vi "Main.vi"(11 "Module Admin":refnum<class "Delacor_lib_QMH_Cloneable Module Admin.lvclass">) -> ()   [LabVIEW 2020, in "Interfase.lvlib"]
doc: "This template is based off of the Queued Message Handler design pattern and the Queued Message Handler project template that ships with LabVIEW.\n\nThe main difference is that the queue is private to this module and communication between modules is performed via Broadcast and Request events.\n\nRequest events are wrapped in public API methods and are handled in the Event Handling Loop (EHL) of this VI. Any module can register for Broadcast events sent by this module. The EHL generates messages based on user interface actions.\n\nThe Message Handling Loop (MHL) processes messages generated by the EHL, or by other messages. The messages are string values, so new messages can be added easily to the Message Cases case structure in the MHL. Each message cluster can also provide an optional value for Message Data, which is a variant that can be converted to whatever message-specific data is required.\n_____\nBased on Delacor QMH Project Template 5.0.0.82."
uses:
  Interfase.lvlib
  <vilib>/Delacor/Delacor QMH/Libraries/Cloneable Module Admin_class/Delacor_lib_QMH_Cloneable Module Admin.lvclass
  C:/Program Files/National Instruments/LabVIEW 2020/vi.lib/Delacor/Delacor QMH/Libraries/Module Admin_class/Delacor_lib_QMH_Module Admin.lvclass
  Controles/Brand combobox.ctl
  Module Data--cluster.ctl
  <vilib>/Delacor/Delacor QMH/Libraries/Cloneable Module Admin_class/Delacor_lib_QMH_Cloneable Module Admin.lvclass/Delacor_lib_QMH_Cloneable Module Admin.ctl
  Stop Argument--cluster.ctl
  <vilib>/Delacor/Delacor QMH/Libraries/Message Queue_class/Delacor_lib_QMH_Message Queue.lvclass/Delacor_lib_QMH_Message Queue.ctl
  <vilib>/Delacor/Delacor QMH/Libraries/Module Admin_class/Delacor_lib_QMH_Module Admin.lvclass/Delacor_lib_QMH_Module Admin.ctl
  Read ADC Argument--cluster.ctl
  Set Port Status Argument--cluster.ctl
  Get Port Status Argument--cluster.ctl
  Set Pin Argument--cluster.ctl
  Get Pin Status Argument--cluster.ctl
  Implementations/Simulado/Simulado.lvclass
  C:/Users/deLili/Desktop/UDLSB IET/701/Instrumentacion Virtual/Fork/Proyecto 7mo/Proyecto-7mo-IV/Abstract/Serial device/Serial device.lvclass
  Implementations/NXP/NXP.lvclass
  Implementations/Cypress/Cypress.lvclass
  <vilib>/Delacor/Delacor QMH/Libraries/Cloneable Module Admin_class/Delacor_lib_QMH_Get Module ID.vi
  <vilib>/Delacor/Delacor QMH/Libraries/Message Queue_class/Delacor_lib_QMH_Enqueue Message (Single).vi
  <vilib>/Delacor/Delacor QMH/Libraries/Module Admin_class/Delacor_lib_QMH_Get External Launch.vi
  <vilib>/Utility/error.llb/Error Cluster From Error Code.vi
  <vilib>/ErrorRing/Error Ring.xnode
  <vilib>/Delacor/Delacor QMH/Libraries/Message Queue_class/Delacor_lib_QMH_Message Queue.lvclass
  Abstract/Serial device/Serial device.lvclass
panel:
  in  "Visa Com Port":refnum<visa-resource-name>
  in  "Serial Device Brand":T1
  in  "Configure serial device":bool
  out "RESPUESTA":string
  in  "Get Pin":bool
  out "Pin Value":bool
  in  "Pin":dbl
  in  "Port":dbl
  in  "Set Port":bool
  in  "Value":string
  in  "Port":dbl
  in  "Get Port":bool
  out "Port Value":bool[](array[boolean])
  in  "Port":dbl
  in  "Set Pin":bool
  in  "Value":bool
  in  "Pin":dbl
  in  "Port":dbl
  in  "Read ADC":bool
  out "error out":errorcluster
  in  "Channel":dbl
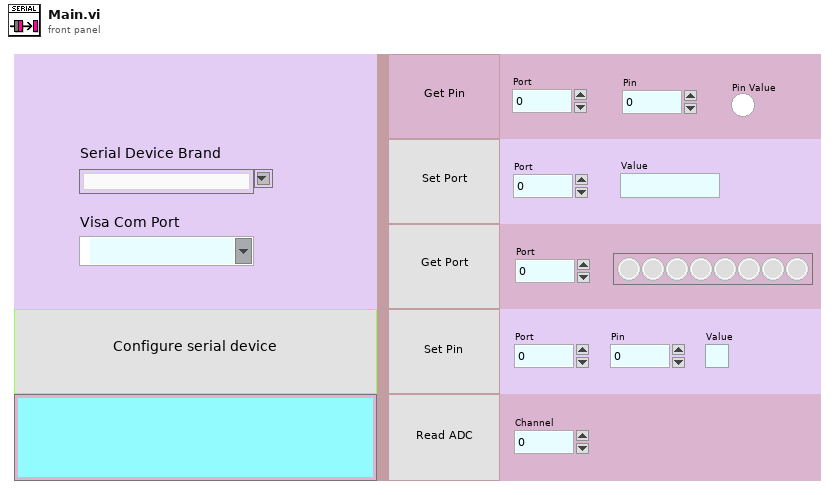
[diagram p1: front panel]
types:
  T1 = typedef "Serial device.lvclass/Brand combobox.ctl" = string
  T2 = typedef "Interfase.lvlib/Request Events--cluster.ctl" = cluster{"Stop Module":refnum<user-event>, "Show Panel":refnum<user-event>, "Hide Panel":refnum<user-event>, "Show Diagram":refnum<user-event>, "Get Module Execution Status":refnum<user-event>, "Read ADC":refnum<user-event>, "Set Port Status":refnum<user-event>, "Get Port Status":refnum<user-event>, "Set Pin":refnum<user-event>, "Get Pin Status":refnum<user-event>}
  T3 = typedef "Interfase.lvlib/Module Data--cluster.ctl" = cluster{"Status":string}
  T4 = enum32{"invalid lock state", "Not Locked", "Locked (No Password)", "Password-protected"}
  T5 = typedef "Interfase.lvlib/Stop Argument--cluster.ctl" = cluster{"Module ID":i32, "Origin":string, "Exit via Stop Module Req?":bool, "Wait for Module to stop?":bool}
  T6 = typedef "Interfase.lvlib/Read ADC Argument--cluster.ctl" = cluster{"Module ID":i32, "Channel":dbl}
  T7 = typedef "Interfase.lvlib/Set Port Status Argument--cluster.ctl" = cluster{"Module ID":i32, "Port":dbl, "Value":string}
  T8 = typedef "Interfase.lvlib/Get Port Status Argument--cluster.ctl" = cluster{"Module ID":i32, "Port":dbl}
  T9 = typedef "Interfase.lvlib/Set Pin Argument--cluster.ctl" = cluster{"Module ID":i32, "Port":dbl, "Pin":dbl, "Value":bool}
  T10 = typedef "Interfase.lvlib/Get Pin Status Argument--cluster.ctl" = cluster{"Module ID":i32, "Port":dbl, "Pin":dbl, "Pin Value":bool}
  T11 = enum32{"Invalid", "Standard", "Closed", "Hidden", "Minimized", "Maximized"}
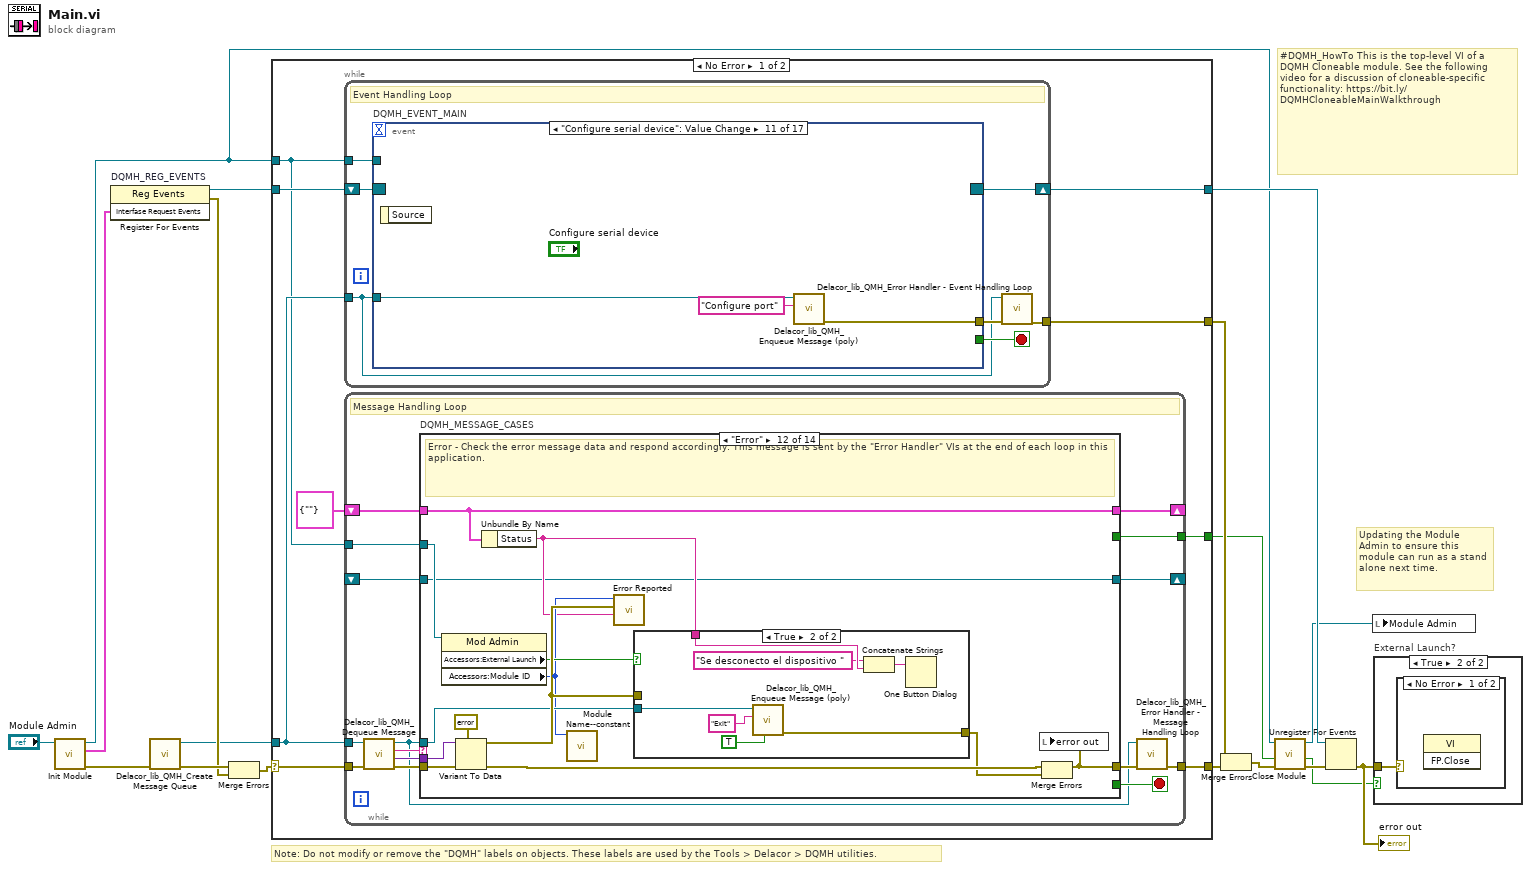
[diagram p0: block diagram]
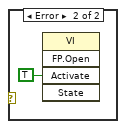
[diagram p3: hidden frame]
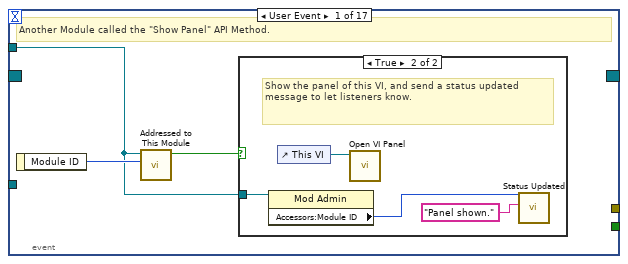
[diagram p4: hidden frame]
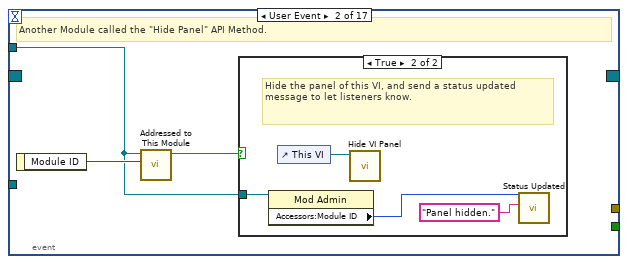
[diagram p6: hidden frame]
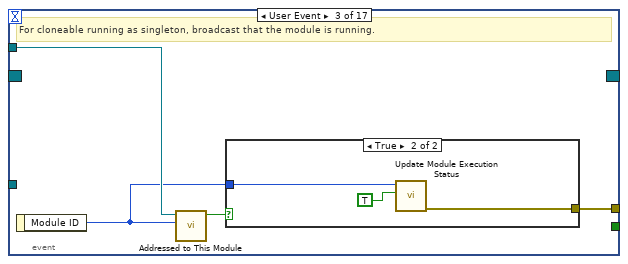
[diagram p8: hidden frame]
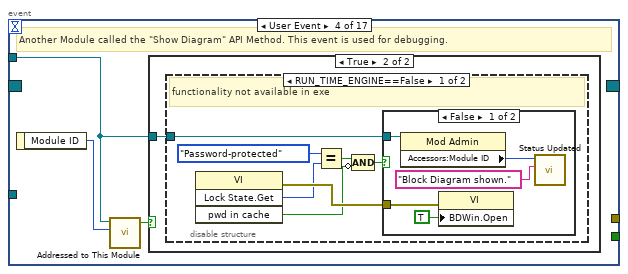
[diagram p10: hidden frame]
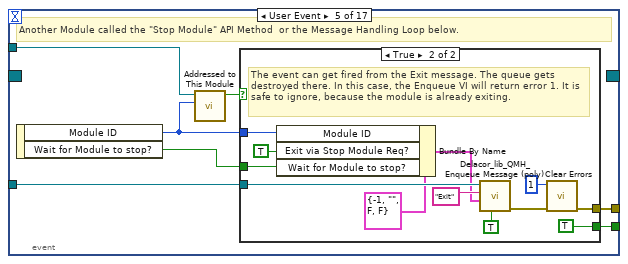
[diagram p14: hidden frame]
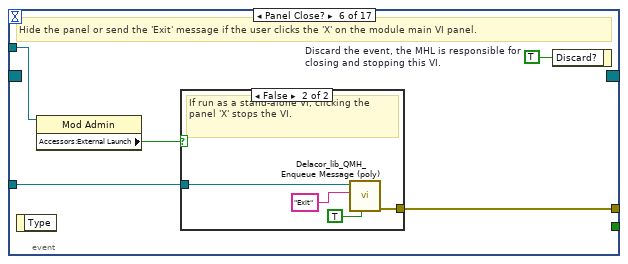
[diagram p16: hidden frame]
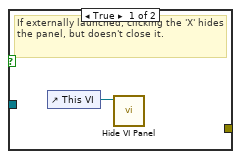
[diagram p17: hidden frame]
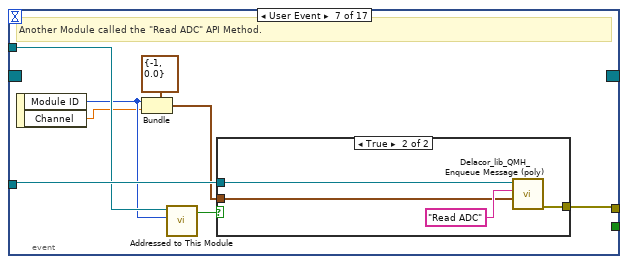
[diagram p18: hidden frame]
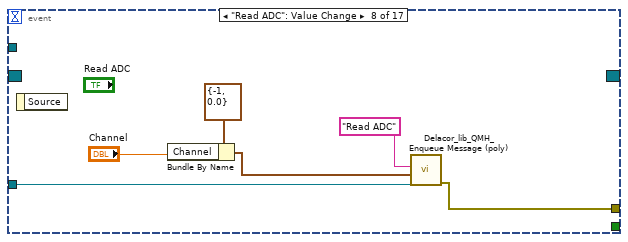
[diagram p20: hidden frame]
diagram:
  # "#DQMH_HowTo This is the top-level VI of a DQMH Cloneable module. See the following video for a discussion of cloneable-specific functionality: https://bit.ly/DQMHCloneableMainWalkthrough"
  # "Note: Do not modify or remove the \"DQMH\" labels on objects. These labels are used by the Tools > Delacor > DQMH utilities."
  # "Updating the Module Admin to ensure this module can run as a stand alone next time."
  n1 = call "Init Module.vi"("Cloneable Module Admin in"="Module Admin") -> ("error out"=w15:errorcluster, "Interfase Request Events"=w7:T2, "Cloneable Module Admin out"=w4:refnum<class "Delacor_lib_QMH_Cloneable Module Admin.lvclass">)  [unwired: 8 in]
  n2 = register-events "DQMH_REG_EVENTS"(w7) -> (reference out=w8:refnum<event-registration>, error out=w10:errorcluster)  [unwired: 2 in]
  n3 = call <vilib>:"Delacor_lib_QMH_Create Message Queue.vi"("error in (no error)"=w15) -> ("error out"=w12:errorcluster, "Message Queue"=w6:refnum<class "Delacor_lib_QMH_Message Queue.lvclass">)  [unwired: 9 in]
  n4 = Merge Errors(w12, w10) -> (w11:errorcluster)
  n5 = case shown="No Error" w11 {
    selector: w11 -> [w25 w419]
    tunnel: [w27 w418] -> w16
    tunnel: [w24 w426] -> w9
    tunnel: w8 -> [w22 w426]
    tunnel: w6 -> [w21 w417]
    tunnel: [w26 _] -> w17
    tunnel: w4 -> [w20 w422]
    tunnel: [w19 _] -> w2
    frame No Error {
      n6 = while {
        tunnel: w21 -> [w28]
        shift-right: [w31] -> w24
        shift-left: w22 -> [w32]
        tunnel: [w33] -> w26
        tunnel: w20 -> [w29]
        stop <- w30 stop-if-true
        # "Event Handling Loop"
        n7 = event "DQMH_EVENT_MAIN" shown="[10] \"Configure serial device\": Value Change" {
          selector: w32 -> [_ _ _ _ _ _ _ _ _ _ _ _ _ _ _ _ _]
          dyn-events: [_ _ _ _ _ _ _ _ _ _ _ _ _ _ _ _ _] -> w31
          timeout: _ -> [_ _ _ _ _ _ _ _ _ _ _ _ _ _ _ _ _]
          tunnel: [_ _ _ _ w74 _ _ _ _ _ _ _ _ _ _ _ _] -> w30
          tunnel: w28 -> [_ _ _ _ w77 w92 w108 w114 w127 w135 w141 w149 w157 w169 w179 w191 w201]
          tunnel: [_ _ w52 _ w78 w95 w101 w113 w119 w132 w140 w142 w156 w160 w180 w182 w196] -> w34
          tunnel: w29 -> [w35 w42 w50 w56 w76 w93 w106 _ w125 _ _ w147 _ w167 _ w189 _]
          event User Event {
            # "Another Module called the \"Show Panel\" API Method."
            n8 = event-data() -> ("Module ID"=w36:i32)  [unwired: 1 in]
            n9 = call "Addressed to This Module.vi"("Module ID from Argument"=w36, "Module Admin"=w35) -> ("Addressed to this instance?"=w37:bool)  [unwired: 8 in, 1 out]
            n10 = case shown="True" w37 {
              tunnel: w35 -> [_ w39]
              frame False {
              }
              frame True {
                # "Show the panel of this VI, and send a status updated message to let listeners know."
                n11 = property class="Mod Admin"(reference=w39) -> ("Accessors:Module ID"=w38:i32)  [unwired: 1 in, 2 out]
                n12 = control-ref of="This VI"() -> (w41:refnum<vi>)
                n13 = call "Open VI Panel.vi"("VI"=w41) -> ()  [unwired: 10 in, 1 out]
                n14 = call "Status Updated.vi"("Status"="Panel shown." ("format string"), "Module ID"=w38) -> ()  [unwired: 9 in, 1 out]
              }
            }
          }
          event User Event {
            # "Another Module called the \"Hide Panel\" API Method."
            n15 = event-data() -> ("Module ID"=w43:i32)  [unwired: 1 in]
            n16 = call "Addressed to This Module.vi"("Module ID from Argument"=w43, "Module Admin"=w42) -> ("Addressed to this instance?"=w44:bool)  [unwired: 8 in, 1 out]
            n17 = case shown="True" w44 {
              tunnel: w42 -> [_ w46]
              frame False {
              }
              frame True {
                # "Hide the panel of this VI, and send a status updated message to let listeners know."
                n18 = property class="Mod Admin"(reference=w46) -> ("Accessors:Module ID"=w45:i32)  [unwired: 1 in, 2 out]
                n19 = control-ref of="This VI"() -> (w48:refnum<vi>)
                n20 = call "Hide VI Panel.vi"("VI"=w48) -> ()  [unwired: 10 in, 1 out]
                n21 = call "Status Updated.vi"("Status"="Panel hidden." ("format string"), "Module ID"=w45) -> ()  [unwired: 9 in, 1 out]
              }
            }
          }
          event User Event {
            # "For cloneable running as singleton, broadcast that the module is running."
            n22 = event-data() -> ("Module ID"=w49:i32)  [unwired: 1 in]
            n23 = call "Addressed to This Module.vi"("Module ID from Argument"=w49, "Module Admin"=w50) -> ("Addressed to this instance?"=w51:bool)  [unwired: 8 in, 1 out]
            n24 = case shown="True" w51 {
              tunnel: [_ w55] -> w52
              tunnel: w49 -> [_ w54]
              frame False {
              }
              frame True {
                n25 = call "Update Module Execution Status.vi"("Running?"=TRUE, "Module ID"=w54) -> ("error out"=w55:errorcluster)  [unwired: 9 in]
              }
            }
          }
          event User Event {
            # "Another Module called the \"Show Diagram\" API Method. This event is used for debugging."
            n26 = event-data() -> ("Module ID"=w57:i32)  [unwired: 1 in]
            n27 = call "Addressed to This Module.vi"("Module ID from Argument"=w57, "Module Admin"=w56) -> ("Addressed to this instance?"=w58:bool)  [unwired: 8 in, 1 out]
            n28 = case shown="True" w58 {
              tunnel: w56 -> [_ w59]
              frame False {
              }
              frame True {
                n29 = disable-structure shown="RUN_TIME_ENGINE==False" {
                  disable-tunnel: w59 -> [w60 _]
                  frame condition #0 (active) {
                    # "functionality not available in exe"
                    n30 = invoke class="VI" method="Lock State.Get"() -> (error out=w66:errorcluster, "Get Lock State"=w65:T4, "pwd in cache"=w62:bool)  [unwired: 4 in, 1 out]
                    n31 = Equal?(x=T4."Password-protected", y=w65) -> (x = y?=w63:bool)
                    n32 = Compound Arithmetic op=AND(w63, invert w62) -> (w61:bool)
                    n33 = case shown="False" w61 {
                      tunnel: w66 -> [w71 _]
                      tunnel: w60 -> [w68 _]
                      frame False {
                        n34 = property class="Mod Admin"(reference=w68) -> ("Accessors:Module ID"=w67:i32)  [unwired: 1 in, 2 out]
                        n35 = property class="VI"(error in=w71, "BDWin.Open"=TRUE ("Block Diagram Window:Open")) -> ()  [unwired: 1 in, 2 out]
                        n36 = call "Status Updated.vi"("Status"="Block Diagram shown." ("format string"), "Module ID"=w67) -> ()  [unwired: 9 in, 1 out]
                      }
                      frame True {
                        # "Password-protected VI, and the password is not in the cache. Do not show the diagram."
                      }
                    }
                  }
                  frame condition #1 {
                  }
                }
              }
            }
          }
          event User Event {
            # "Another Module called the \"Stop Module\" API Method  or the Message Handling Loop below."
            n37 = event-data() -> ("Module ID"=w72:i32, "Wait for Module to stop?"=w73:bool)  [unwired: 1 in]
            n38 = call "Addressed to This Module.vi"("Module ID from Argument"=w72, "Module Admin"=w76) -> ("Addressed to this instance?"=w75:bool)  [unwired: 8 in, 1 out]
            n39 = case shown="True" w75 {
              tunnel: [_ w89] -> w78
              tunnel: w77 -> [_ w85]
              tunnel: [_ TRUE] -> w74
              tunnel: w73 -> [_ w80]
              tunnel: w72 -> [_ w82]
              frame False {
              }
              frame True {
                # "The event can get fired from the Exit message. The queue gets destroyed there. In this case, the Enqueue VI will return error 1. It is safe to ignore, because the module is already exiting."
                n40 = Bundle By Name(cluster=T5 {"Module ID"=-1, "Origin"="", "Exit via Stop Module Req?"=FALSE, "Wait for Module to stop?"=FALSE} ("Stop Argument"), "Module ID"=w82, "Exit via Stop Module Req?"=TRUE, "Wait for Module to stop?"=w80) -> (w79:T5)
                n41 = call-poly <vilib>:"Delacor_lib_QMH_Enqueue Message (poly).vi"("Priority Message? (F)"=TRUE, "Message Data"=w79, "Message"="Exit", "Message Queue in"=w85) -> ("error out"=w90:errorcluster)  [unwired: 6 in, 1 out]
                n42 = call <vilib>:"Clear Errors.vi"("error in (no error)"=w90, "specific error code to clear (0: all)"=1) -> ("error out"=w89:errorcluster)  [unwired: 4 in, 1 out]
              }
            }
          }
          event Panel Close? {
            w94 = TRUE  # Discard the event, the MHL is responsible for closing and stopping this VI.
            # "Hide the panel or send the 'Exit' message if the user clicks the 'X' on the module main VI panel."
            n43 = event-data() -> ()  [unwired: 1 in, 1 out]
            n44 = property class="Mod Admin"(reference=w93) -> ("Accessors:External Launch"=w91:bool)  [unwired: 1 in, 2 out]
            n45 = case shown="False" w91 {
              tunnel: w92 -> [_ w99]
              tunnel: [_ w100] -> w95
              frame True {
                # "If externally launched, clicking the 'X' hides the panel, but doesn't close it."
                n46 = control-ref of="This VI"() -> (w96:refnum<vi>)
                n47 = call "Hide VI Panel.vi"("VI"=w96) -> ()  [unwired: 10 in, 1 out]
              }
              frame False {
                # "If run as a stand-alone VI, clicking the panel 'X' stops the VI."
                n48 = call-poly <vilib>:"Delacor_lib_QMH_Enqueue Message (poly).vi"("Priority Message? (F)"=TRUE, "Message"="Exit", "Message Queue in"=w99) -> ("error out"=w100:errorcluster)  [unwired: 7 in, 1 out]
              }
            }
            n49 = event-data("Discard?"=w94) -> ()  [unwired: 1 in, 1 out]
          }
          event User Event {
            # "Another Module called the \"Read ADC\" API Method."
            n50 = event-data() -> ("Module ID"=w103:i32, "Channel"=w102:dbl)  [unwired: 1 in]
            n51 = Bundle(cluster=T6 {"Module ID"=-1, "Channel"=0.0} ("Read ADC Argument"), "Module ID"=w103, "Channel"=w102) -> (w104:T6)
            n52 = call "Addressed to This Module.vi"("Module ID from Argument"=w103, "Module Admin"=w106) -> ("Addressed to this instance?"=w107:bool)  [unwired: 8 in, 1 out]
            n53 = case shown="True" w107 {
              tunnel: w108 -> [_ w112]
              tunnel: w104 -> [_ w110]
              tunnel: [_ w109] -> w101
              frame False {
              }
              frame True {
                n54 = call-poly <vilib>:"Delacor_lib_QMH_Enqueue Message (poly).vi"("Message Data"=w110, "Message"="Read ADC", "Message Queue in"=w112) -> ("error out"=w109:errorcluster)  [unwired: 7 in, 1 out]
              }
            }
          }
          event "Read ADC": Value Change {
            n55 = event-data() -> ()  [unwired: 1 in, 1 out]
            n56 = Bundle By Name(cluster=T6 {"Module ID"=-1, "Channel"=0.0} ("Read ADC Argument"), "Channel"="Channel") -> (w116:T6)
            n57 = call-poly <vilib>:"Delacor_lib_QMH_Enqueue Message (poly).vi"("Message Data"=w116, "Message"="Read ADC", "Message Queue in"=w114) -> ("error out"=w113:errorcluster)  [unwired: 7 in, 1 out]
          }
          event User Event {
            # "Another Module called the \"Set Port Status\" API Method."
            n58 = event-data() -> ("Module ID"=w122:i32, "Port"=w121:dbl, "Value"=w120:string)  [unwired: 1 in]
            n59 = Bundle(cluster=T7 {"Module ID"=-1, "Port"=0.0, "Value"=""} ("Set Port Status Argument"), "Module ID"=w122, "Port"=w121, "Value"=w120) -> (w123:T7)
            n60 = call "Addressed to This Module.vi"("Module ID from Argument"=w122, "Module Admin"=w125) -> ("Addressed to this instance?"=w126:bool)  [unwired: 8 in, 1 out]
            n61 = case shown="True" w126 {
              tunnel: w127 -> [_ w131]
              tunnel: w123 -> [_ w129]
              tunnel: [_ w128] -> w119
              frame False {
              }
              frame True {
                n62 = call-poly <vilib>:"Delacor_lib_QMH_Enqueue Message (poly).vi"("Message Data"=w129, "Message"="Set Port Status", "Message Queue in"=w131) -> ("error out"=w128:errorcluster)  [unwired: 7 in, 1 out]
              }
            }
          }
          event "Set Port": Value Change {
            n63 = event-data() -> ()  [unwired: 1 in, 1 out]
            n64 = Bundle By Name(cluster=T7 {"Module ID"=-1, "Port"=0.0, "Value"=""} ("Set Port Status Argument"), "Port"="Port", "Value"="Value") -> (w136:T7)
            n65 = call-poly <vilib>:"Delacor_lib_QMH_Enqueue Message (poly).vi"("Message Data"=w136, "Message"="Set Port Status", "Message Queue in"=w135) -> ("error out"=w132:errorcluster)  [unwired: 7 in, 1 out]
          }
          event "Configure serial device": Value Change {
            n66 = event-data() -> ()  [unwired: 1 in, 1 out]
            n67 = call-poly <vilib>:"Delacor_lib_QMH_Enqueue Message (poly).vi"("Message"="Configure port", "Message Queue in"=w141) -> ("error out"=w140:errorcluster)  [unwired: 8 in, 1 out]
          }
          event User Event {
            # "Another Module called the \"Get Port Status\" API Method."
            n68 = event-data() -> ("Module ID"=w144:i32, "Port"=w143:dbl)  [unwired: 1 in]
            n69 = Bundle(cluster=T8 {"Module ID"=-1, "Port"=0.0} ("Get Port Status Argument"), "Module ID"=w144, "Port"=w143) -> (w145:T8)
            n70 = call "Addressed to This Module.vi"("Module ID from Argument"=w144, "Module Admin"=w147) -> ("Addressed to this instance?"=w148:bool)  [unwired: 8 in, 1 out]
            n71 = case shown="True" w148 {
              tunnel: w149 -> [_ w153]
              tunnel: w145 -> [_ w151]
              tunnel: [_ w150] -> w142
              frame False {
              }
              frame True {
                n72 = call-poly <vilib>:"Delacor_lib_QMH_Enqueue Message (poly).vi"("Message Data"=w151, "Message"="Get Port Status", "Message Queue in"=w153) -> ("error out"=w150:errorcluster)  [unwired: 7 in, 1 out]
              }
            }
          }
          event "Get Port": Value Change {
            n73 = event-data() -> ()  [unwired: 1 in, 1 out]
            n74 = Bundle By Name(cluster=T8 {"Module ID"=-1, "Port"=0.0} ("Get Port Status Argument"), "Port"="Port") -> (w155:T8)
            n75 = call-poly <vilib>:"Delacor_lib_QMH_Enqueue Message (poly).vi"("Message Data"=w155, "Message"="Get Port Status", "Message Queue in"=w157) -> ("error out"=w156:errorcluster)  [unwired: 7 in, 1 out]
          }
          event User Event {
            # "Another Module called the \"Set Pin\" API Method."
            n76 = event-data() -> ("Module ID"=w164:i32, "Port"=w163:dbl, "Pin"=w162:dbl, "Value"=w161:bool)  [unwired: 1 in]
            n77 = Bundle(cluster=T9 {"Module ID"=-1, "Port"=0.0, "Pin"=0.0, "Value"=FALSE} ("Set Pin Argument"), "Module ID"=w164, "Port"=w163, "Pin"=w162, "Value"=w161) -> (w165:T9)
            n78 = call "Addressed to This Module.vi"("Module ID from Argument"=w164, "Module Admin"=w167) -> ("Addressed to this instance?"=w168:bool)  [unwired: 8 in, 1 out]
            n79 = case shown="True" w168 {
              tunnel: w169 -> [_ w173]
              tunnel: w165 -> [_ w171]
              tunnel: [_ w170] -> w160
              frame False {
              }
              frame True {
                n80 = call-poly <vilib>:"Delacor_lib_QMH_Enqueue Message (poly).vi"("Message Data"=w171, "Message"="Set Pin", "Message Queue in"=w173) -> ("error out"=w170:errorcluster)  [unwired: 7 in, 1 out]
              }
            }
          }
          event "Set Pin": Value Change {
            n81 = event-data() -> ()  [unwired: 1 in, 1 out]
            n82 = Bundle By Name(cluster=T9 {"Module ID"=-1, "Port"=0.0, "Pin"=0.0, "Value"=FALSE} ("Set Pin Argument"), "Port"="Port", "Pin"="Pin", "Value"="Value") -> (w177:T9)
            n83 = call-poly <vilib>:"Delacor_lib_QMH_Enqueue Message (poly).vi"("Message Data"=w177, "Message"="Set Pin", "Message Queue in"=w179) -> ("error out"=w180:errorcluster)  [unwired: 7 in, 1 out]
          }
          event User Event {
            # "Another Module called the \"Get Pin Status\" API Method."
            n84 = event-data() -> ("Module ID"=w186:i32, "Port"=w185:dbl, "Pin"=w184:dbl, "Pin Value"=w183:bool)  [unwired: 1 in]
            n85 = Bundle(cluster=T10 {"Module ID"=-1, "Port"=0.0, "Pin"=0.0, "Pin Value"=FALSE} ("Get Pin Status Argument"), "Module ID"=w186, "Port"=w185, "Pin"=w184, "Pin Value"=w183) -> (w187:T10)
            n86 = call "Addressed to This Module.vi"("Module ID from Argument"=w186, "Module Admin"=w189) -> ("Addressed to this instance?"=w190:bool)  [unwired: 8 in, 1 out]
            n87 = case shown="True" w190 {
              tunnel: w191 -> [_ w195]
              tunnel: w187 -> [_ w193]
              tunnel: [_ w192] -> w182
              frame False {
              }
              frame True {
                n88 = call-poly <vilib>:"Delacor_lib_QMH_Enqueue Message (poly).vi"("Message Data"=w193, "Message"="Get Pin Status", "Message Queue in"=w195) -> ("error out"=w192:errorcluster)  [unwired: 7 in, 1 out]
              }
            }
          }
          event "Get Pin": Value Change {
            n89 = event-data() -> ()  [unwired: 1 in, 1 out]
            n90 = Bundle By Name(cluster=T10 {"Module ID"=-1, "Port"=0.0, "Pin"=0.0, "Pin Value"=FALSE} ("Get Pin Status Argument"), "Port"="Port", "Pin"="Pin") -> (w197:T10)
            n91 = call-poly <vilib>:"Delacor_lib_QMH_Enqueue Message (poly).vi"("Message Data"=w197, "Message"="Get Pin Status", "Message Queue in"=w201) -> ("error out"=w196:errorcluster)  [unwired: 7 in, 1 out]
          }
        }
        n92 = call-dynamic "Delacor_lib_QMH_Error Handler - Event Handling Loop.vi"("error in (no error)"=w34, "Message Queue in"=w28) -> ("dup error in"=w33:errorcluster)  [unwired: 8 in, 1 out]
      }
      n93 = while {
        tunnel: w21 -> [w208]
        shift-right: [w212] -> _
        shift-left: T3 {"Status"=""} ("Data Cluster") -> [w213]
        tunnel: w25 -> [w216]
        tunnel: [w214] -> w27
        tunnel: w20 -> [w206]
        tunnel: [w205] -> w19
        shift-right: [w204] -> _
        shift-left: _ -> [w203]
        stop <- w211 stop-if-true
        # "Message Handling Loop"
        n94 = call-dynamic "Delacor_lib_QMH_Dequeue Message.vi"("error in (no error)"=w216, "Message Queue in"=w208) -> ("error out"=w215:errorcluster, "Message Data"=w209:variant, "Message"=w210:string, "Message Queue out"=w207:refnum<class "Delacor_lib_QMH_Message Queue.lvclass">)  [unwired: 6 in]
        n95 = case "DQMH_MESSAGE_CASES" shown="\"Error\"" w210 {
          selector: w210 -> [_ _ _ _ _ _ _ _ _ _ _ _ _ w404]
          tunnel: w207 -> [_ _ _ w255 _ w282 _ w321 _ _ _ w360 w393 _]
          tunnel: w215 -> [w234 w244 w253 w270 w277 w295 w312 w331 w348 w352 w355 w368 w399 w406]
          tunnel: [w232 w244 w253 w257 w275 w285 w301 w319 w336 w351 w355 w364 w396 w407] -> w217
          tunnel: w213 -> [w225 w240 w252 w269 w276 w294 w311 w330 w347 w350 w354 w358 w392 w405]
          tunnel: [w225 w239 w252 w269 w276 w294 w311 w330 w347 w350 w354 w358 w392 w405] -> w212
          tunnel: [_ _ _ _ _ _ _ _ _ _ _ _ w391 _] -> w211
          tunnel: w209 -> [_ _ _ w268 w274 w292 w309 w328 w345 _ _ w363 w389 _]
          tunnel: w206 -> [w220 _ _ _ _ _ _ _ _ _ _ w362 w385 w402]
          tunnel: [_ _ _ _ _ _ _ _ _ _ _ _ w387 _] -> w205
          tunnel: [w218 w237 w251 w254 w271 w281 w303 w323 w340 w349 w353 w356 w382 w400] -> w204
          tunnel: w203 -> [w218 _ w251 w265 w271 w289 w305 w322 w341 w349 w353 w356 w383 w400]
          frame "Initialize" {
            # "Initialize - Any operation that needs to be done before the module can receive messages. Synchronize Caller Events.vi will inform Start Module.vi that the module has launched and is ready to receive messages. Module Did Init.vi will broadcast that the module initialized."
            n96 = call "Synchronize Caller Events.vi"("error in (no error)"=w234, "Module Admin"=w220) -> ("error out"=w233:errorcluster, "Module Admin out"=w219:refnum<class "Delacor_lib_QMH_Cloneable Module Admin.lvclass">)  [unwired: 8 in]
            n97 = property class="Mod Admin"(reference=w219) -> ("Accessors:Module ID"=w222:i32, "Accessors:External Launch"=w221:bool)  [unwired: 1 in, 2 out]
            n98 = call "Module Name--constant.vi"("Module ID"=w222) -> ("Module Name"=w229:string)  [unwired: 10 in]
            n99 = property class="VI"("Front Panel.Title"=w229) -> (reference out=w231:refnum<vi>, error out=w236:errorcluster)  [unwired: 2 in]
            n100 = Select(t=T11."Hidden" ("State"), s=w221, f=T11."Standard" ("State")) -> (s? t:f=w226:T11)
            n101 = invoke class="VI" method="FP.Open"(reference=w231, error in=w236, "State"=w226) -> (reference out=w230:refnum<vi>, error out=w235:errorcluster)  [unwired: 2 in, 3 out]
            n102 = call "Module Name--constant.vi"("Module ID"=w222) -> ("Module Name"=w223:string)  [unwired: 10 in]
            n103 = invoke class="VI" method="FP.Center"(reference=w230, error in=w235) -> ()  [unwired: 1 in, 3 out]
            n104 = call "Module Did Init.vi"("error in (no error)"=w233, "Initialized?"=TRUE, "Origin"=w223, "Module ID"=w222) -> ("error out"=w232:errorcluster)  [unwired: 7 in]
          }
          frame "Configure port" {
            n105 = case shown="\"CY\"" "Serial Device Brand" {
              tunnel: [refnum<class "Simulado.lvclass"> refnum ("Simulado.lvclass") refnum<class "NXP.lvclass"> refnum ("NXP.lvclass") refnum<class "Cypress.lvclass"> refnum ("Cypress.lvclass")] -> w243
              tunnel: ["SD" "NX" "CY"] -> w242
              frame "SD", Default {
              }
              frame "NX" {
              }
              frame "CY" {
              }
            }
            n106 = call-dynamic "Initialize.vi"("VISA Com Port"="Visa Com Port", "Serial Device Brand"=w242, "Serial device in"=w243) -> ("Serial device out"=w237:refnum<class "Serial device.lvclass">)  [unwired: 7 in, 1 out]
            n107 = Bundle By Name(cluster=w240, "Status"="Serial Device Brand") -> (w239:T3)
          }
          frame "--- Module Specific ---" {
            # "Separator -- The following cases handle messages specific to this Module."
          }
          frame "Read ADC" {
            n108 = Variant To Data(error in=w270, type=T6 {"Module ID"=-1, "Channel"=0.0} ("Read ADC Argument"), Variant=w268) -> (data=w266:T6, error out=w258:errorcluster)
            n109 = Unbundle By Name(w266) -> ("Channel"=w263:dbl)
            n110 = call-dynamic "Read ADC.vi"("ADC canal"=w263, "Serial device in"=w265) -> ("error out"=w262:errorcluster, "Serial device out"=w264:refnum<class "Serial device.lvclass">)  [unwired: 8 in]
            n111 = call-dynamic "Read ADC Response.vi"("error in (no error)"=w262, "Serial device in"=w264) -> ("error out"=w259:errorcluster, "Buffer"=w261:string, "Serial device out"=w254:refnum<class "Serial device.lvclass">)  [unwired: 7 in]
            n112 = call-poly <vilib>:"Delacor_lib_QMH_Enqueue Message (poly).vi"("error in (no error)"=w259, "Message Data"=w261, "Message"="Respuesta del micro", "Message Queue in"=w255) -> ("error out"=w256:errorcluster)  [unwired: 6 in, 1 out]
            n113 = Merge Errors(w256, w258) -> (w257:errorcluster)
          }
          frame "Respuesta del micro" {
            n114 = Variant To Data(error in=w277, type="", Variant=w274) -> (data=→"RESPUESTA":string, error out=w275:errorcluster)
          }
          frame "Set Port Status" {
            n115 = Variant To Data(error in=w295, type=T7 {"Module ID"=-1, "Port"=0.0, "Value"=""} ("Set Port Status Argument"), Variant=w292) -> (data=w290:T7, error out=w293:errorcluster)
            n116 = Unbundle By Name(w290) -> ("Port"=w279:dbl, "Value"=w278:string)
            n117 = call-dynamic "Set Port Status.vi"("Value"=w278, "Port"=w279, "Serial device in"=w289) -> ("error out"=w287:errorcluster, "Serial device out"=w288:refnum<class "Serial device.lvclass">)  [unwired: 7 in]
            n118 = call-dynamic "Read ADC Response.vi"("error in (no error)"=w287, "Serial device in"=w288) -> ("error out"=w286:errorcluster, "Buffer"=w280:string, "Serial device out"=w281:refnum<class "Serial device.lvclass">)  [unwired: 7 in]
            n119 = call-poly <vilib>:"Delacor_lib_QMH_Enqueue Message (poly).vi"("error in (no error)"=w286, "Message Data"=w280, "Message"="Respuesta del micro", "Message Queue in"=w282) -> ("error out"=w284:errorcluster)  [unwired: 6 in, 1 out]
            n120 = Merge Errors(w284, w293) -> (w285:errorcluster)
          }
          frame "Get Port Status" {
            n121 = Variant To Data(error in=w312, type=T8 {"Module ID"=-1, "Port"=0.0} ("Get Port Status Argument"), Variant=w309) -> (data=w307:T8, error out=w310:errorcluster)
            n122 = Unbundle By Name(w307) -> ("Port"=w306:dbl)
            n123 = call-dynamic "Get Port Status.vi"("Port"=w306, "Serial device in"=w305) -> ("error out"=w300:errorcluster, "Serial device out"=w304:refnum<class "Serial device.lvclass">)  [unwired: 8 in]
            n124 = call-dynamic "Get Port Status Response.vi"("error in (no error)"=w300, "Serial device in"=w304) -> ("error out"=w299:errorcluster, "Response"=w302:string, "Serial device out"=w303:refnum<class "Serial device.lvclass">)  [unwired: 7 in]
            n125 = Hexadecimal String To Number(string=w302) -> (number=w298:u32)  [unwired: 2 in, 1 out]
            n126 = Merge Errors(w299, w310) -> (w301:errorcluster)
            n127 = Number To Boolean Array(number=w298) -> (Boolean array=w297:bool[])
            n128 = Reverse 1D Array(array=w297) -> (reversed array=→"Port Value":bool[])
          }
          frame "Set Pin" {
            n129 = Variant To Data(error in=w331, type=T9 {"Module ID"=-1, "Port"=0.0, "Pin"=0.0, "Value"=FALSE} ("Set Pin Argument"), Variant=w328) -> (data=w326:T9, error out=w329:errorcluster)
            n130 = Unbundle By Name(w326) -> ("Port"=w315:dbl, "Pin"=w314:dbl, "Value"=w313:bool)
            n131 = call-dynamic "Set Pin Status.vi"("Serial device in"=w322, "Port"=w315, "Pin"=w314, "Value"=w313) -> ("Serial device out"=w325:refnum<class "Serial device.lvclass">, "error out"=w324:errorcluster)  [unwired: 10 in]
            n132 = call-dynamic "Read ADC Response.vi"("error in (no error)"=w324, "Serial device in"=w325) -> ("error out"=w320:errorcluster, "Buffer"=w316:string, "Serial device out"=w323:refnum<class "Serial device.lvclass">)  [unwired: 7 in]
            n133 = call-poly <vilib>:"Delacor_lib_QMH_Enqueue Message (poly).vi"("error in (no error)"=w320, "Message Data"=w316, "Message"="Respuesta del micro", "Message Queue in"=w321) -> ("error out"=w318:errorcluster)  [unwired: 6 in, 1 out]
            n134 = Merge Errors(w318, w329) -> (w319:errorcluster)
          }
          frame "Get Pin Status" {
            n135 = Variant To Data(error in=w348, type=T10 {"Module ID"=-1, "Port"=0.0, "Pin"=0.0, "Pin Value"=FALSE} ("Get Pin Status Argument"), Variant=w345) -> (data=w343:T10, error out=w346:errorcluster)
            n136 = Unbundle By Name(w343) -> ("Port"=w338:dbl, "Pin"=w337:dbl)
            n137 = call-dynamic "Get Pin Status.vi"("Pin"=w337, "Port"=w338, "Serial device in"=w341) -> ("error out"=w342:errorcluster, "Serial device out"=w339:refnum<class "Serial device.lvclass">)  [unwired: 7 in]
            n138 = call-dynamic "Get Pin Status Response.vi"("error in (no error)"=w342, "Serial device in"=w339) -> ("Value"=w335:string, "Serial device out"=w340:refnum<class "Serial device.lvclass">)  [unwired: 7 in, 1 out]
            n139 = Decimal String To Number(string=w335) -> (number=w334:i32)  [unwired: 2 in, 1 out]
            n140 = Equal To 0?(x=w334) -> (x = 0?=w333:bool)
            n141 = Merge Errors(w346) -> (w336:errorcluster)
            n142 = Not(x=w333) -> (.not. x?=→"Pin Value":bool)
          }
          frame "---Copy This Frame---" {
            # "Duplicate this frame when creating new messages.  Change this comment in the duplicated frame to describe this message."
            n143 = Merge Errors(w352) -> (w351:errorcluster)
          }
          frame "--- Exit and Error Handling---" {
            # "Separator - the following cases handle errors and exit messages."
          }
          frame "Error" {
            # "Error - Check the error message data and respond accordingly. This message is sent by the \"Error Handler\" VIs at the end of each loop in this application."
            n144 = property class="Mod Admin"(reference=w362) -> ("Accessors:External Launch"=w361:bool, "Accessors:Module ID"=w359:i32)  [unwired: 1 in, 2 out]
            n145 = Variant To Data(error in=w368, type=errorcluster {"status"=FALSE, "code"=0, "source"=""} ("error constant"), Variant=w363) -> (data=w369:errorcluster, error out=w366:errorcluster)
            n146 = Unbundle By Name(w358) -> ("Status"=w357:string)
            n147 = call "Module Name--constant.vi"("Module ID"=w359) -> ()  [unwired: 10 in, 1 out]
            n148 = call "Error Reported.vi"("Additional Information"=w357, "Error"=w369, "Module ID"=w359) -> ()  [unwired: 8 in, 1 out]
            n149 = case shown="True" w361 {
              tunnel: [w374 w375] -> w365
              tunnel: w360 -> [w372 w376]
              tunnel: w369 -> [w373 _]
              tunnel: w357 -> [_ w381]
              frame False {
                n150 = call <vilib>:"Simple Error Handler.vi"("error in (no error)"=w373) -> ()  [unwired: 4 in, 5 out]
                n151 = call-poly <vilib>:"Delacor_lib_QMH_Enqueue Message (poly).vi"("Priority Message? (F)"=TRUE, "Message"="Exit", "Message Queue in"=w372) -> ("error out"=w374:errorcluster)  [unwired: 7 in, 1 out]
              }
              frame True {
                n152 = call-poly <vilib>:"Delacor_lib_QMH_Enqueue Message (poly).vi"("Priority Message? (F)"=TRUE, "Message"="Exit", "Message Queue in"=w376) -> ("error out"=w375:errorcluster)  [unwired: 7 in, 1 out]
                n153 = Concatenate Strings("Se desconecto el dispositivo " ("string"), w381) -> (w379:string)
                n154 = One Button Dialog(message=w379) -> ()  [unwired: 1 in, 1 out]
              }
            }
            n155 = Merge Errors(w366, w365) -> (w364:errorcluster)
            n156 = local write "error out"(w364) -> ()
          }
          frame "Exit" {
            w390 = 91  # 91: not all Exit messages will have an argument
            w391 = TRUE  # Stop the VI
            # "Release the message queue reference"
            # "Exit - Exit the application."
            n157 = Variant To Data(error in=w399, type=T5 {"Module ID"=-1, "Origin"="", "Exit via Stop Module Req?"=FALSE, "Wait for Module to stop?"=FALSE} ("Stop Argument"), Variant=w389) -> (data=w386:T5, error out=w394:errorcluster)
            n158 = call <vilib>:"Clear Errors.vi"("error in (no error)"=w394, "specific error code to clear (0: all)"=w390) -> ("error out"=w398:errorcluster)  [unwired: 4 in, 1 out]
            n159 = control-ref of="This VI"() -> (w384:refnum<vi>)
            n160 = call-dynamic "Close Connection.vi"("Serial device in"=w383) -> ("Serial device out"=w382:refnum<class "Serial device.lvclass">)  [unwired: 9 in, 1 out]
            n161 = call-dynamic "Delacor_lib_QMH_Release Message Queue.vi"("error in (no error)"=w398, "Message Queue"=w393) -> ("error out"=w397:errorcluster)  [unwired: 9 in]
            n162 = call "Handle Exit.vi"("Stop Argument"=w386, "Module Admin in"=w385, "VI reference"=w384) -> ("error out"=w395:errorcluster, "Wait for Stop?"=w387:bool)  [unwired: 7 in]
            n163 = Merge Errors(w397, w395) -> (w396:errorcluster)
          }
          frame Default {
            # "'Default' case only runs if there is a message that isn't defined in any of the other cases.  Output a programming error."
            n164 = property class="Mod Admin"(reference=w402) -> ("Accessors:Module ID"=w401:i32)  [unwired: 1 in, 2 out]
            n165 = call "Module Name--constant.vi"("Module ID"=w401) -> ("Module Name"=w403:string)  [unwired: 10 in]
            n166 = xnode "Error Ring"("parameter 0"=w404, "parameter 1"=w403) -> ("error out"=w408:errorcluster)
            n167 = Merge Errors(w406, w408) -> (w407:errorcluster)
          }
        }
        n168 = call-dynamic "Delacor_lib_QMH_Error Handler - Message Handling Loop.vi"("error in (no error)"=w217, "Message Queue in"=w207) -> ("dup error in"=w214:errorcluster)  [unwired: 8 in, 1 out]
      }
    }
    frame Error {
      n169 = call "Synchronize Caller Events.vi"("Module Admin"=w422) -> ("Module Admin out"=w421:refnum<class "Delacor_lib_QMH_Cloneable Module Admin.lvclass">)  [unwired: 9 in, 1 out]
      n170 = property class="Mod Admin"(reference=w421) -> ("Accessors:Module ID"=w420:i32)  [unwired: 1 in, 2 out]
      n171 = call-dynamic "Delacor_lib_QMH_Release Message Queue.vi"("error in (no error)"=w419, "Message Queue"=w417) -> ("error out"=w418:errorcluster)  [unwired: 9 in]
      n172 = call "Module Name--constant.vi"("Module ID"=w420) -> ("Module Name"=w425:string)  [unwired: 10 in]
      n173 = Format Into String(format string="An error occurred during initialization. %s is no longer running.", w425) -> (resulting string=w423:string)  [unwired: 2 in, 1 out]
      n174 = call "Error Reported.vi"("Additional Information"=w423, "Error"=w418, "Module ID"=w420) -> ()  [unwired: 8 in, 1 out]
    }
  }
  n175 = Merge Errors(w17, w16) -> (w18:errorcluster)
  n176 = call "Close Module.vi"("error in"=w18, "Wait for stop?"=w2, "Module Admin in"=w4) -> ("error out"=w14:errorcluster, "External Launch"=w1:bool, "Module Admin out"=w3:refnum<class "Delacor_lib_QMH_Cloneable Module Admin.lvclass">)  [unwired: 6 in]
  n177 = Unregister For Events(event registration refnum=w9, error in=w14) -> (error out=w13:errorcluster)
  "error out" <- w13
  n178 = local write "Module Admin"(w3) -> ()
  n179 = case "External Launch?" shown="True" w1 {
    tunnel: w13 -> [_ w427]
    frame False {
    }
    frame True {
      n180 = case shown="No Error" w427 {
        frame No Error {
          n181 = invoke class="VI" method="FP.Close"() -> ()  [unwired: 3 in, 3 out]
        }
        frame Error {
          n182 = invoke class="VI" method="FP.Open"("Activate"=TRUE ("Activate?")) -> ()  [unwired: 4 in, 5 out]
        }
      }
    }
  }
